vi "Apply special move.vi"(8 "error in (no error)":errorcluster, 10 "Position in":refnum<class "Position.lvclass">, 11 "Promotion in":refnum<class "Promotion.lvclass">) -> (0 "error out":errorcluster, 2 "Position out":refnum<class "Position.lvclass">, 3 "Promotion out":refnum<class "Promotion.lvclass">)   [LabVIEW 2016, in "Chesslib.lvlib" / "Promotion.lvclass"]
uses:
  Promotion.lvclass
  C:/Users/GRTaggJ/Documents/Projects/checkmate/Chesslib/Moves/Move/Move.lvclass
  Position/Position.lvclass
  Move/Move.lvclass/Move.ctl
  Pieces/Piece/Piece.lvclass/Piece.ctl
  Promotion.lvclass/Promotion.ctl
  typedef/Piece type.ctl
  Pieces/Piece/Piece.lvclass
  Move/Move.lvclass
  Chesslib.lvlib
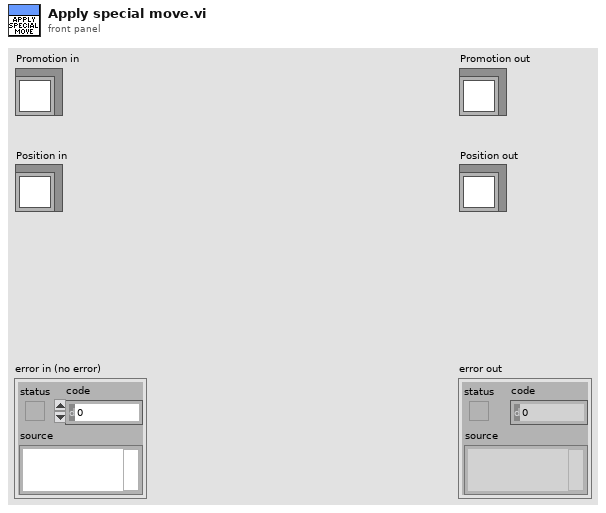
[diagram p1: front panel]
types:
  T1 = typedef "Chesslib.lvlib/Promotion.lvclass/Promotion piece.ctl" = enum16{"Bishop", "Knight", "Rook", "Queen"}
  T2 = typedef "Chesslib.lvlib/Piece type.ctl" = enum16{"Pawn", "Bishop", "Knight", "Rook", "Queen", "King"}
  T3 = typedef "Chesslib.lvlib/Square.ctl" = cluster{"File":T4, "Rank":T5}
  T4 = typedef "Chesslib.lvlib/File.ctl" = enum8{"a", "b", "c", "d", "e", "f", "g", "h"}
  T5 = typedef "Chesslib.lvlib/Rank.ctl" = enum8{"1", "2", "3", "4", "5", "6", "7", "8"}
  T6 = typedef "Chesslib.lvlib/Color.ctl" = enum16{"White", "Black"}
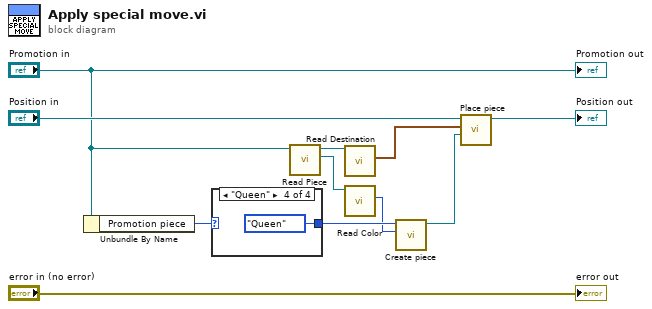
[diagram p0: block diagram]
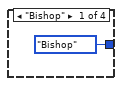
[diagram p2: hidden frame]
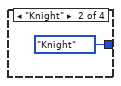
[diagram p3: hidden frame]
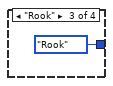
[diagram p4: hidden frame]
diagram:
  n1 = Unbundle By Name("Promotion in") -> ("Promotion piece"=w6:T1)
  n2 = case shown="\"Queen\"" w6 {
    tunnel: [Piece_type."Bishop" ("Piece type") Piece_type."Knight" ("Piece type") Piece_type."Rook" ("Piece type") Piece_type."Queen" ("Piece type")] -> w5
    frame "Bishop" {
    }
    frame "Knight" {
    }
    frame "Rook" {
    }
    frame "Queen" {
    }
  }
  n3 = call "Read Piece.vi"("Move in"="Promotion in") -> ("Chesslib.lvlib:Piece.lvclass"=w8:refnum<class "Piece.lvclass">, "Move out"=w7:refnum<class "Promotion.lvclass">)  [unwired: 9 in]
  n4 = call "Read Destination.vi"("Move in"=w7) -> ("Square"=w2:T3)  [unwired: 9 in, 1 out]
  n5 = call "Read Color.vi"("Piece in"=w8) -> ("Color"=w4:T6)  [unwired: 10 in]
  n6 = call "Create piece.vi"("Piece color"=w4, "Piece type"=w5) -> ("Piece out"=w1:refnum<class "Piece.lvclass">)  [unwired: 9 in]
  n7 = call "Place piece.vi"("Piece"=w1, "Destination"=w2, "Position in"="Position in") -> ("Position out"=→"Position out":refnum<class "Position.lvclass">)  [unwired: 7 in, 1 out]
  "error out" <- "error in (no error)"
  "Promotion out" <- "Promotion in"
